vi "Disconnect OPC UA.vi"(8 "error in":errorcluster, 10 "subscription IDs":T1[](array[typedef])) -> (0 "error out":errorcluster)   [LabVIEW 2021]
uses:
  <vilib>/OPCUA/controls/Subscription ID.ctl
  <vilib>/OPCUA/controls/OPC UA Client Refnum.ctl
  <vilib>/OPCUA/NI OPC UA Client.lvlib
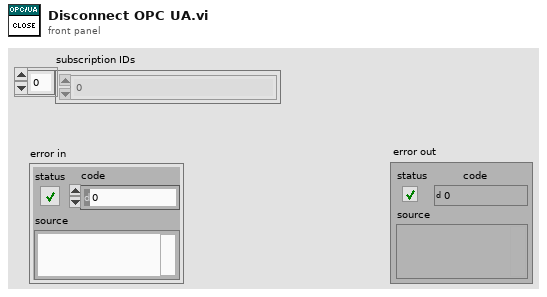
[diagram p1: front panel]
types:
  T1 = typedef "Subscription ID.ctl" = u32
  T2 = typedef "OPC UA Client Refnum.ctl" = refnum<k21>
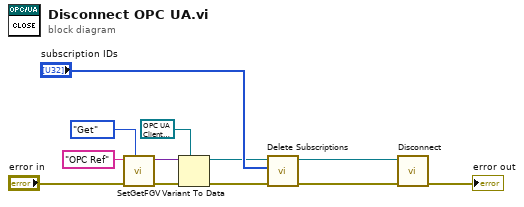
[diagram p0: block diagram]
diagram:
  n1 = call "SetGetFGV.vi"("Method (Get)"=enum16{"Get", "Set"}."Get", "error in"="error in", "Name"="OPC Ref") -> ("error out"=w4:errorcluster, "Data out"=w8:variant)  [unwired: 7 in]
  n2 = Variant To Data(error in=w4, type=T2 refnum ("OPC UA client refnum out"), Variant=w8) -> (data=w2:T2, error out=w3:errorcluster)
  n3 = call <vilib>:"Delete Subscriptions.vi"("error in (no error)"=w3, "subscription IDs"="subscription IDs", "OPC UA client refnum in"=w2) -> ("error out"=w10:errorcluster, "OPC UA client refnum out"=w9:T2)  [unwired: 6 in, 1 out]
  n4 = call <vilib>:"Disconnect.vi"("error in (no error)"=w10, "OPC UA client refnum in"=w9) -> ("error out"=→"error out":errorcluster)  [unwired: 9 in]
